vi "NumberPositionAreaRobot.vi"(7 "EventsRef":refnum<class "Events.lvclass">, 8 "error in (no error)":errorcluster, 9 "position(x,y)":dbl[](array[numeric]), 10 "Field":refnum<class "Field.lvclass">, 11 "Utilities in":refnum<class "Utilities.lvclass">) -> (0 "error out":errorcluster, 1 "NumericArea":i32, 3 "Utilities out":refnum<class "Utilities.lvclass">)   [LabVIEW 2021, in "Utilities.lvclass"]
uses:
  Utilities.lvclass
  Field_class/Field.lvclass
  Events_class/Events.lvclass
  Events_class/Events.lvclass/Events.ctl
  Events_class/Read ball_inside_enemy_goalie_area.vi
  Events_class/Read ball_inside_our_goalie_area.vi
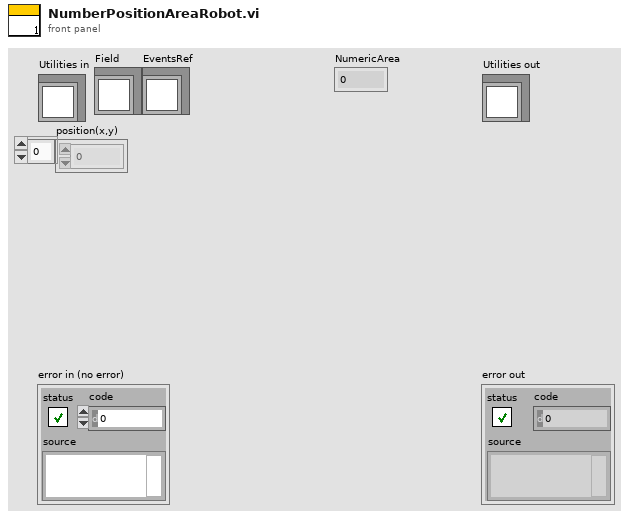
[diagram p1: front panel]
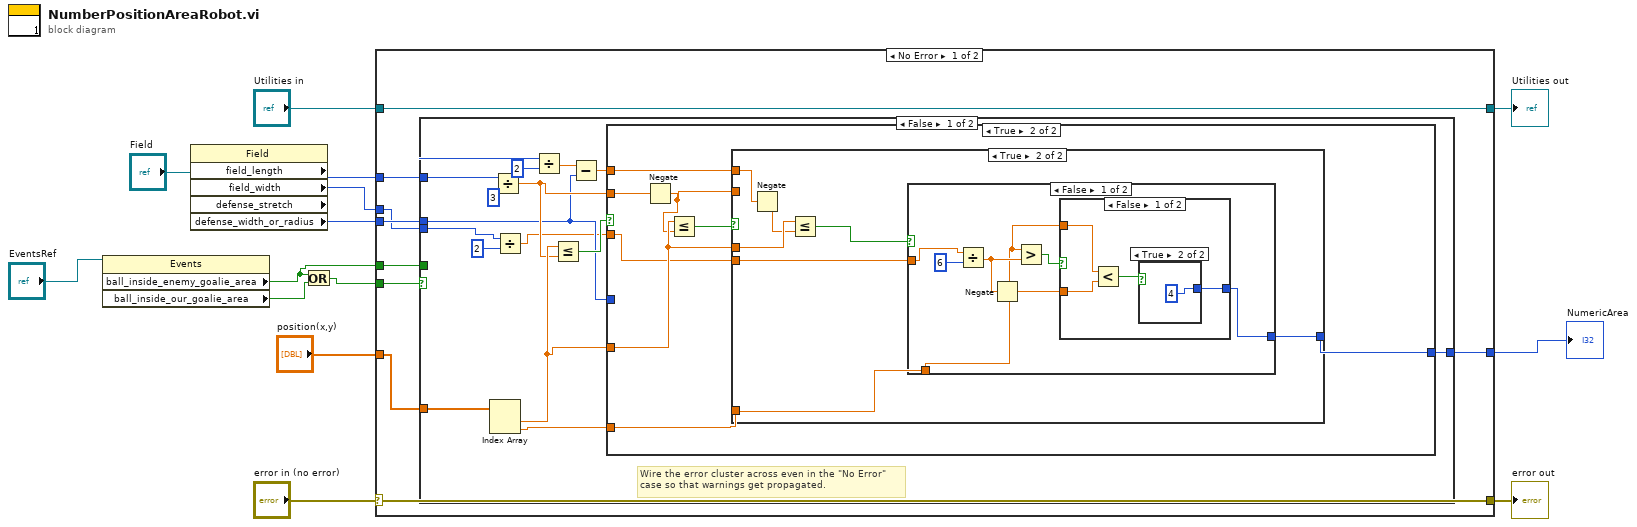
[diagram p0: block diagram]
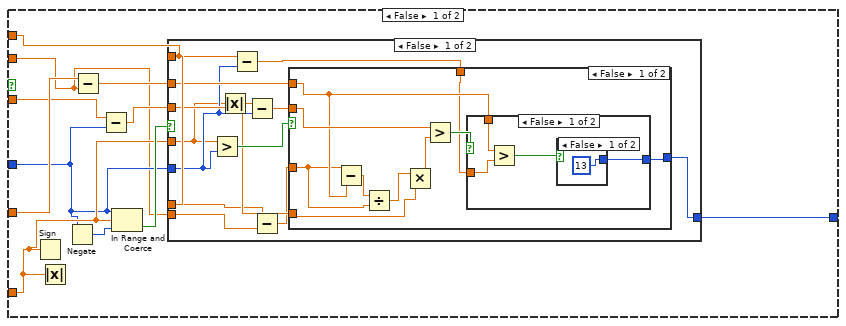
[diagram p2: hidden frame]
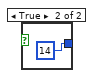
[diagram p3: hidden frame]
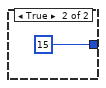
[diagram p4: hidden frame]
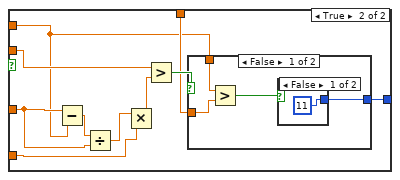
[diagram p5: hidden frame]
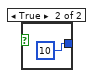
[diagram p6: hidden frame]
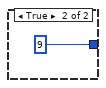
[diagram p7: hidden frame]
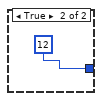
[diagram p8: hidden frame]
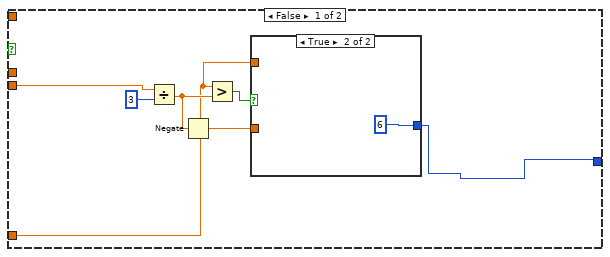
[diagram p9: hidden frame]
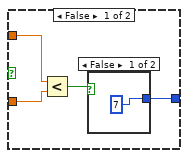
[diagram p10: hidden frame]
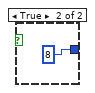
[diagram p11: hidden frame]
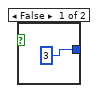
[diagram p12: hidden frame]
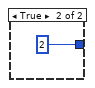
[diagram p13: hidden frame]
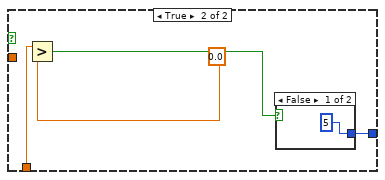
[diagram p14: hidden frame]
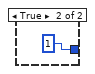
[diagram p15: hidden frame]
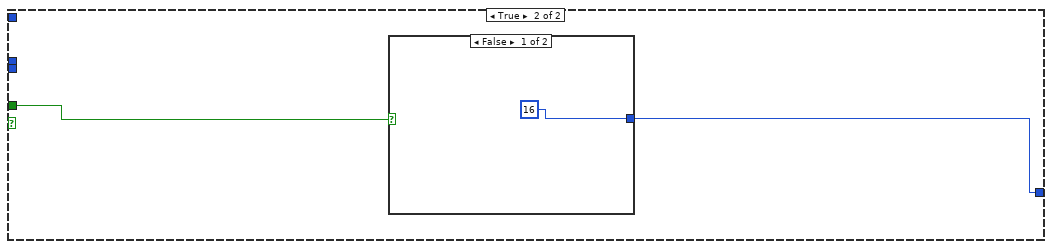
[diagram p16: hidden frame]
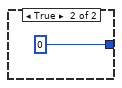
[diagram p17: hidden frame]
diagram:
  n1 = property class="Events"(reference="EventsRef") -> ("ball_inside_enemy_goalie_area"=w2:bool, "ball_inside_our_goalie_area"=w4:bool)  [unwired: 1 in, 2 out]
  n2 = property class="Field" props=["field_length", "field_width", "defense_stretch", "defense_width_or_radius"](reference="Field") -> ("field_length"=w8:i32, "field_width"=w6:i32, "defense_width_or_radius"=w7:i32)  [unwired: 1 in, 3 out]
  n3 = Or(x=w2, y=w4) -> (x .or. y?=w3:bool)
  n4 = case shown="No Error" "error in (no error)" {
    selector: "error in (no error)" -> [w22 w152]
    tunnel: [w22 w152] -> w13
    tunnel: [w23 w151] -> w11
    tunnel: "Utilities in" -> [w23 w151]
    tunnel: "position(x,y)" -> [w21 _]
    tunnel: w8 -> [w20 _]
    tunnel: w7 -> [w19 _]
    tunnel: w6 -> [w18 _]
    tunnel: w3 -> [w17 _]
    tunnel: w2 -> [w16 _]
    tunnel: [w15 _] -> w1
    frame No Error {
      n5 = case shown="False" w17 {
        tunnel: w21 -> [w36 _]
        tunnel: w20 -> [w33 _]
        tunnel: w19 -> [w27 _]
        tunnel: w18 -> [w26 _]
        tunnel: w16 -> [_ w148]
        tunnel: [w28 w147] -> w15
        frame False {
          # "Wire the error cluster across even in the \"No Error\"\ncase so that warnings get propagated."
          n6 = Index Array(array=w36) -> (element #1=w35:dbl, element #2=w29:dbl)  [unwired: 2 in]
          n7 = Divide(x=w33, y=3 ("field_length")) -> (x/y=w34:dbl)
          n8 = Divide(x=w26, y=2) -> (x/y=w24:dbl)
          n9 = Divide(x=w33, y=2) -> (x/y=w31:dbl)
          n10 = Less Or Equal?(x=w35, y=w34) -> (x <= y?=w37:bool)
          n11 = Subtract(x=w31, y=w27) -> (x-y=w30:dbl)
          n12 = case shown="True" w37 {
            tunnel: w35 -> [w49 w103]
            tunnel: w34 -> [w40 w105]
            tunnel: w30 -> [w39 w102]
            tunnel: w29 -> [w45 w101]
            tunnel: [w46 w100] -> w28
            tunnel: w27 -> [w42 _]
            tunnel: w24 -> [w43 w98]
            frame False {
              n13 = Sign(1:w45) -> ()  [unwired: 1 out]
              n14 = Absolute Value(x=w45) -> ()  [unwired: 1 out]
              n15 = Negate(x=w42) -> (-x=w48:i32)
              n16 = Subtract(x=w49, y=w40) -> (x-y=w44:dbl)
              n17 = Subtract(x=w43, y=w42) -> (x-y=w41:dbl)
              n18 = In Range and Coerce(upper limit=w42, x=w45, lower limit=w48) -> (In Range?=w47:bool)  [unwired: 1 out]
              n19 = case shown="False" w47 {
                tunnel: [w55 12] -> w46
                tunnel: w45 -> [w50 _]
                tunnel: w42 -> [w53 _]
                tunnel: w44 -> [w61 _]
                tunnel: w41 -> [w60 _]
                tunnel: w39 -> [w58 _]
                tunnel: w40 -> [w57 _]
                tunnel: w39 -> [w54 _]
                frame False {
                  n20 = Greater?(x=w50, y=w53) -> (0:w62:bool)
                  n21 = Absolute Value(x=w50) -> (abs(x)=w51:dbl)
                  n22 = Subtract(x=w54, y=w53) -> (x-y=w52:dbl)
                  n23 = Subtract(x=w51, y=w53) -> (x-y=w59:dbl)
                  n24 = Subtract(x=w58, y=w57) -> (x-y=w56:dbl)
                  n25 = case shown="False" w62 {
                    tunnel: w61 -> [w67 w80]
                    tunnel: w60 -> [w65 w86]
                    tunnel: w59 -> [w68 w84]
                    tunnel: w56 -> [w66 w88]
                    tunnel: [w63 w82] -> w55
                    tunnel: w52 -> [w64 w81]
                    frame False {
                      n26 = Subtract(x=w66, y=w67) -> (x-y=w69:dbl)
                      n27 = Divide(x=w69, y=w66) -> (x/y=w70:dbl)
                      n28 = Multiply(x=w70, y=w65) -> (x*y=w71:dbl)
                      n29 = Greater?(x=w68, y=w71) -> (0:w72:bool)
                      n30 = case shown="False" w72 {
                        tunnel: [w73 15] -> w63
                        tunnel: w64 -> [w76 _]
                        tunnel: w67 -> [w75 _]
                        frame False {
                          n31 = Greater?(x=w75, y=w76) -> (0:w74:bool)
                          n32 = case shown="False" w74 {
                            tunnel: [13 14] -> w73
                            frame False {
                            }
                            frame True {
                            }
                          }
                        }
                        frame True {
                        }
                      }
                    }
                    frame True {
                      n33 = Subtract(x=w88, y=w80) -> (x-y=w89:dbl)
                      n34 = Divide(x=w89, y=w88) -> (x/y=w87:dbl)
                      n35 = Multiply(x=w87, y=w86) -> (x*y=w85:dbl)
                      n36 = Greater?(x=w84, y=w85) -> (0:w83:bool)
                      n37 = case shown="False" w83 {
                        tunnel: [w90 9] -> w82
                        tunnel: w81 -> [w93 _]
                        tunnel: w80 -> [w92 _]
                        frame False {
                          n38 = Greater?(x=w92, y=w93) -> (0:w91:bool)
                          n39 = case shown="False" w91 {
                            tunnel: [11 10] -> w90
                            frame False {
                            }
                            frame True {
                            }
                          }
                        }
                        frame True {
                        }
                      }
                    }
                  }
                }
                frame True {
                }
              }
            }
            frame True {
              n40 = Negate(x=w105) -> (-x=w99:dbl)
              n41 = Less Or Equal?(x=w103, y=w99) -> (x <= y?=w104:bool)
              n42 = case shown="True" w104 {
                tunnel: w103 -> [_ w126]
                tunnel: w102 -> [_ w125]
                tunnel: w101 -> [w108 w122]
                tunnel: [w107 w121] -> w100
                tunnel: w99 -> [_ _]
                tunnel: w98 -> [w106 w120]
                frame False {
                  n43 = Divide(x=w106, y=3) -> (x/y=w110:dbl)
                  n44 = Negate(x=w110) -> (-x=w109:dbl)
                  n45 = Greater?(x=w108, y=w110) -> (0:w111:bool)
                  n46 = case shown="True" w111 {
                    tunnel: [w113 6] -> w107
                    tunnel: w108 -> [w116 _]
                    tunnel: w109 -> [w115 _]
                    frame False {
                      n47 = Less?(x=w116, y=w115) -> (x < y?=w114:bool)
                      n48 = case shown="False" w114 {
                        tunnel: [7 8] -> w113
                        frame False {
                        }
                        frame True {
                        }
                      }
                    }
                    frame True {
                    }
                  }
                }
                frame True {
                  n49 = Negate(x=w125) -> (-x=w124:dbl)
                  n50 = Less Or Equal?(x=w126, y=w124) -> (x <= y?=w123:bool)
                  n51 = case shown="False" w123 {
                    tunnel: w122 -> [w129 w144]
                    tunnel: [w128 w141] -> w121
                    tunnel: w120 -> [w127 _]
                    frame False {
                      n52 = Divide(x=w127, y=6) -> (x/y=w131:dbl)
                      n53 = Negate(x=w131) -> (-x=w130:dbl)
                      n54 = Greater?(x=w129, y=w131) -> (0:w132:bool)
                      n55 = case shown="False" w132 {
                        tunnel: [w134 2] -> w128
                        tunnel: w129 -> [w137 _]
                        tunnel: w130 -> [w136 _]
                        frame False {
                          n56 = Less?(x=w137, y=w136) -> (x < y?=w135:bool)
                          n57 = case shown="True" w135 {
                            tunnel: [3 4] -> w134
                            frame False {
                            }
                            frame True {
                            }
                          }
                        }
                        frame True {
                        }
                      }
                    }
                    frame True {
                      n58 = Greater?(x=w144, y=0.0) -> (0:w142:bool)
                      n59 = case shown="False" w142 {
                        tunnel: [5 1] -> w141
                        frame False {
                        }
                        frame True {
                        }
                      }
                    }
                  }
                }
              }
            }
          }
        }
        frame True {
          n60 = case shown="False" w148 {
            tunnel: [16 0] -> w147
            frame False {
            }
            frame True {
            }
          }
        }
      }
    }
    frame Error {
    }
  }
  "error out" <- w13
  "Utilities out" <- w11
  "NumericArea" <- w1
